vi "Win32 GetBestRoute.vi"(8 "error in (no error)":errorcluster, 11 "address":refnum<class "IPv4 Network Address.lvclass">) -> (0 "error out":errorcluster, 2 "pBestRoute":u32[](array[numeric]))   [LabVIEW 2020, in "NI_WFCN.lvlib" / "IPv4 Network Address.lvclass"]
doc: "Win32: Call GetBestRoute() to determine if an IPv4 address is routable."
uses:
  <vilib>/net/WFCN/Addressing/IPv4 Network Address/IPv4 Network Address.lvclass
  <vilib>/net/WFCN/Addressing/IPv4 Network Address/IPv4 Network Address.lvclass/IPv4 Network Address.ctl
  <vilib>/net/WFCN/NI_WFCN.lvlib
  iphlpapi.dll
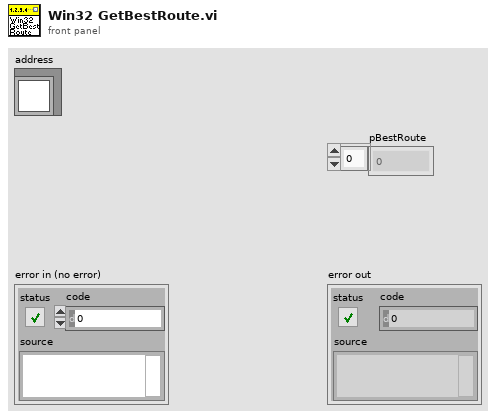
[diagram p1: front panel]
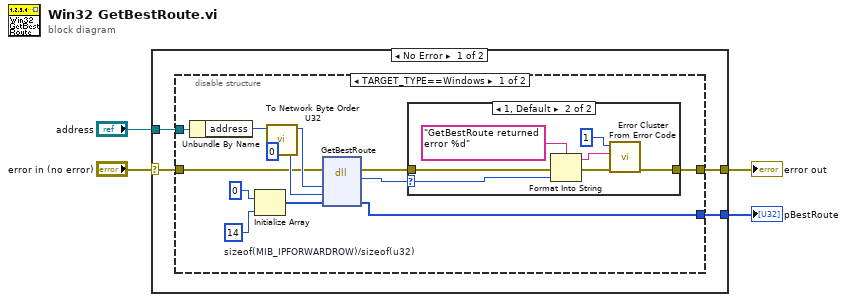
[diagram p0: block diagram]
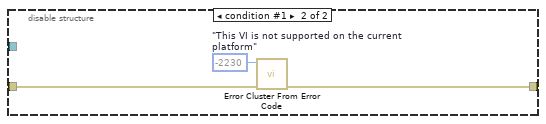
[diagram p3: hidden frame]
diagram:
  n1 = case shown="No Error" "error in (no error)" {
    selector: "error in (no error)" -> [w6 w32]
    tunnel: "address" -> [w8 _]
    tunnel: [w7 w32] -> w4
    tunnel: [w5 _] -> w1
    frame No Error {
      n2 = disable-structure shown="TARGET_TYPE==Windows" {
        disable-tunnel: w8 -> [w16 _]
        disable-tunnel: w6 -> [w14 w30]
        disable-tunnel: [w11 w29] -> w7
        disable-tunnel: [w9 _] -> w5
        frame condition #0 (active) {
          w19 = 14  # sizeof(MIB_IPFORWARDROW)/sizeof(u32)
          n3 = Unbundle By Name(w16) -> ("address"=w10:u32)
          n4 = Initialize Array(u32 0, w19) -> (w18:u32[])
          n5 = call <vilib>:"To Network Byte Order U32.vi"("network byte order"=w10) -> ("native byte order"=w17:u32)  [unwired: 6 in]
          n6 = dll-call lib="iphlpapi.dll" fn="GetBestRoute"(error in=w14, "dwBestAddr"=w17, "dwSourceAddr"=u32 0, "pBestRoute"=w18) -> (error out=w12:errorcluster, "return type"=w13:i32, "pBestRoute"=w9:u32[])  [unwired: 4 in, 1 out]
          n7 = case shown="1, Default" w13 {
            selector: w13 -> [_ w24]
            tunnel: w12 -> [w21 w26]
            tunnel: [w21 w28] -> w11
            frame 0 {
            }
            frame 1, Default {
              n8 = Format Into String(format string="GetBestRoute returned error %d", error in=w26, w24) -> (resulting string=w22:string, error out=w23:errorcluster)  [unwired: 1 in]
              n9 = call <vilib>:"Error Cluster From Error Code.vi"("error in (no error)"=w23, "error message (\"\")"=w22, "error code (0)"=1) -> ("error out"=w28:errorcluster)  [unwired: 6 in]
            }
          }
        }
        frame condition #1 {
          w31 = -2230  # "This VI is not supported on the current platform"
          n10 = call <vilib>:"Error Cluster From Error Code.vi"("error in (no error)"=w30, "error code (0)"=w31) -> ("error out"=w29:errorcluster)  [unwired: 7 in]
        }
      }
    }
    frame Error {
    }
  }
  "error out" <- w4
  "pBestRoute" <- w1
